vi "Synchio.Shutdown.vi"(8 "error in (no error)":errorcluster, 10 "AIAO Tasks":T1={"AI task"=["", ""], "AO Task"=[""]}, 11 "SynchIO.USB4431 in":refnum<class "SynchIO.USB4431.lvclass">) -> (0 "error out":errorcluster, 3 "SynchIO.USB4431 out":refnum<class "SynchIO.USB4431.lvclass">)   [LabVIEW 2016, in "SynchIO.USB4431.lvclass"]
uses:
  SynchIO.USB4431.lvclass
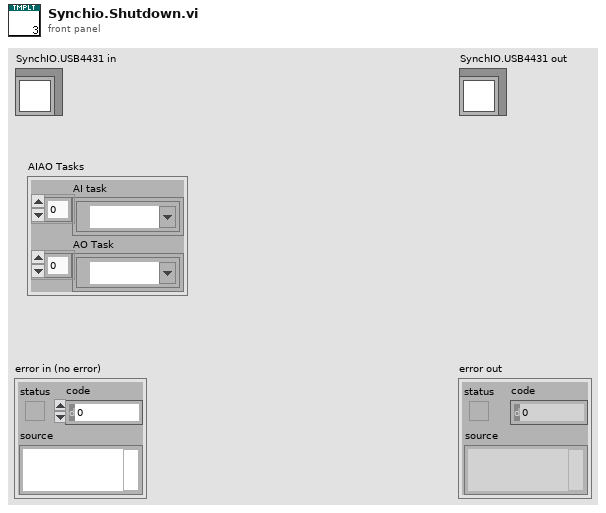
[diagram p1: front panel]
types:
  T1 = cluster{"AI task":refnum<k21>[], "AO Task":refnum<k21>[]}
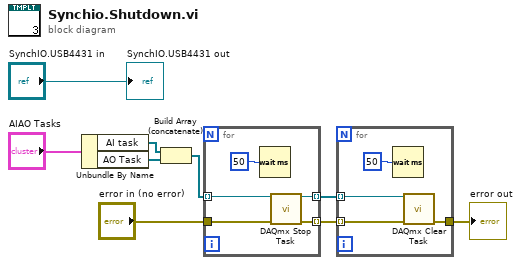
[diagram p0: block diagram]
diagram:
  n1 = Unbundle By Name("AIAO Tasks") -> ("AI task"=w4:refnum<k21>[], "AO Task"=w3:refnum<k21>[])
  n2 = Build Array (concatenate)(w4, w3) -> (w7:refnum<k21>[])
  n3 = for {
    tunnel: [w14] -> w9 mode=indexing
    tunnel: [w13] -> w8 mode=indexing
    tunnel: w7 -> [w10] mode=indexing
    tunnel: "error in (no error)" -> [w11]
    n4 = Wait (ms)(milliseconds to wait=u32 50) -> ()  [unwired: 1 out]
    n5 = call <vilib>:"DAQmx Stop Task.vi"("task/channels in"=w10, "error in"=w11) -> ("task out"=w14:refnum<k21>, "error out"=w13:errorcluster)  [unwired: 12 in]
  }
  n6 = for {
    tunnel: w9 -> [w18] mode=indexing
    tunnel: w8 -> [w17] mode=indexing
    tunnel: [w15] -> w5
    n7 = Wait (ms)(milliseconds to wait=u32 50) -> ()  [unwired: 1 out]
    n8 = call <vilib>:"DAQmx Clear Task.vi"("task in"=w18, "error in"=w17) -> ("error out"=w15:errorcluster)  [unwired: 13 in]
  }
  "error out" <- w5
  "SynchIO.USB4431 out" <- "SynchIO.USB4431 in"
